vi "Keithley 2002 Arm Config.vi"(0 "GPIB address":string="16", 1 "Hours":string="12", 2 "Minutes":string="00", 3 "Seconds":string="00", 4 "async input (line 2:1)":u16(ring)=1 items=["line 1", "line 2", "line 3", "line 4", "line 5", "line 6"], 5 "count (set:0)":u16(ring) items=["set  value", "infinite", "min", "max"], 6 "async output (line 1:0)":u16(ring) items=["line 1", "line 2", "line 3", "line 4", "line 5", "line 6"], 7 "count value":dbl=1.0 min=1.0 max=99999.0 step=1.0, 8 "direction":bool, 9 "source (imm:1)":u16(ring)=1 items=["hold", "immediate", "manual", "bus", "trigger link", "external", "Real-Time Clock"], 11 "error in":T1, 12 "Year":string="1994", 13 "Month":string="08", 14 "Day":string="01") -> (15 "error out":T1)   [LabVIEW 2020]
doc: "This VI is used to configure the settings for the Arm Layer of the trigger model. The model consists of 3 layers, the Arm Layer, the Scan Layer (Arm2), and the Measure Layer (Trigger).\n\nIn general, the instrument requires an arm event to allow operation to proceed to the next layer (Arm2)."
panel:
  # "source\nacceptor"
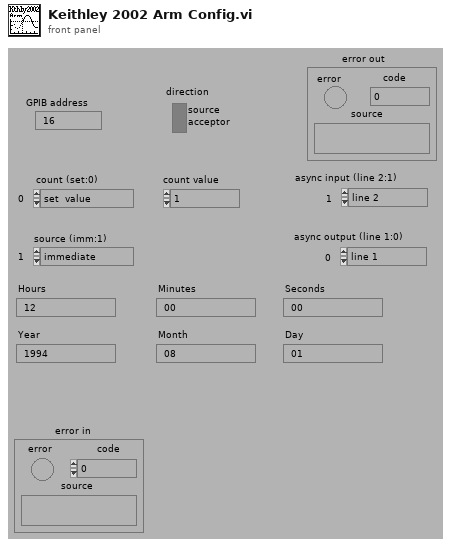
[diagram p1: front panel]
types:
  T1 = cluster{"error":bool, "code":i32, "source":string}
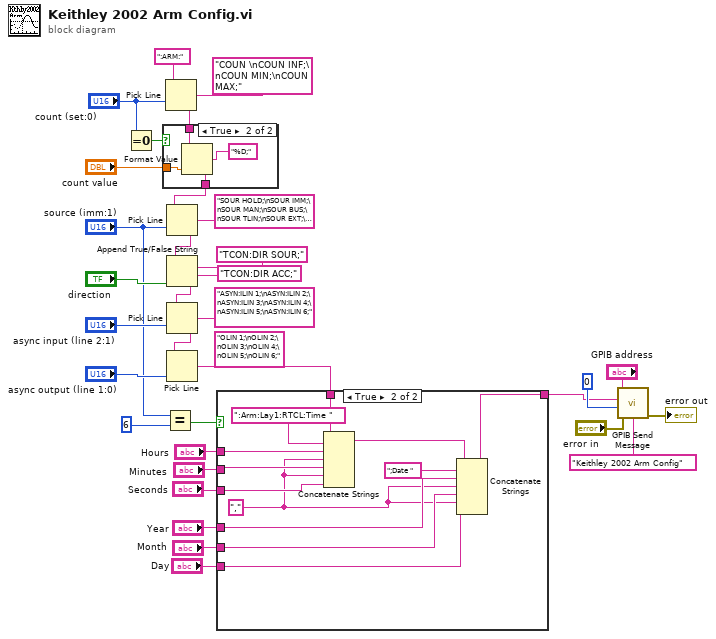
[diagram p0: block diagram]
diagram:
  n1 = Equal To 0?(x="count (set:0)") -> (x = 0?=w25:bool)
  n2 = Equal?(x="source (imm:1)", y=6) -> (x = y?=w9:bool)
  n3 = Pick Line(string ("")=":ARM:", multi-line string="COUN \nCOUN INF;\nCOUN MIN;\nCOUN MAX;", line index="count (set:0)") -> (output string=w26:string)
  n4 = case shown="True" w25 {
    tunnel: "count value" -> [_ w39]
    tunnel: w26 -> [w35 w38]
    tunnel: [w35 w36] -> w24
    frame False {
    }
    frame True {
      n5 = Format Value(string ("")=w38, format string="%D;", value (0)=w39) -> (output string=w36:string)
    }
  }
  n6 = Pick Line(string ("")=w24, multi-line string="SOUR HOLD;\nSOUR IMM;\nSOUR MAN;\nSOUR BUS;\nSOUR TLIN;\nSOUR EXT;\nSour RTCL;", line index="source (imm:1)") -> (output string=w21:string)
  n7 = Append True/False String(1:"direction", 2:"TCON:DIR ACC;", 3:"TCON:DIR SOUR;", 4:w21) -> (0:w13:string)
  n8 = Pick Line(string ("")=w13, multi-line string="ASYN:ILIN 1;\nASYN:ILIN 2;\nASYN:ILIN 3;\nASYN:ILIN 4;\nASYN:ILIN 5;\nASYN:ILIN 6;", line index="async input (line 2:1)") -> (output string=w15:string)
  n9 = Pick Line(string ("")=w15, multi-line string="OLIN 1;\nOLIN 2;\nOLIN 3;\nOLIN 4;\nOLIN 5;\nOLIN 6;", line index="async output (line 1:0)") -> (output string=w1:string)
  n10 = case shown="True" w9 {
    tunnel: "Hours" -> [_ w51]
    tunnel: "Minutes" -> [_ w50]
    tunnel: "Seconds" -> [_ w49]
    tunnel: "Year" -> [_ w47]
    tunnel: "Month" -> [_ w46]
    tunnel: "Day" -> [_ w44]
    tunnel: [w40 w43] -> w2
    tunnel: w1 -> [w40 w42]
    frame False {
    }
    frame True {
      w45 = ","
      n11 = Concatenate Strings(w42, ":Arm:Lay1:RTCL:Time ", w51, w45, w50, w45, w49) -> (w41:string)
      n12 = Concatenate Strings(w41, ";Date ", w47, w45, w46, w45, w44) -> (w43:string)
    }
  }
  n13 = call "GPIB Send Message.vi"("address string"="GPIB address", "write buffer"=w2, "source"="Keithley 2002 Arm Config", "write mode (set END:0)"=0, "error in"="error in") -> ("error out"=→"error out":T1)  [unwired: 2 in, 2 out]
